vi "EZ430-Chronos - Read Accelerometer.vi"() -> ()   [LabVIEW 2011, in "LVH-EZ430.lvlib"]
doc: "This example demonstrates how to read the accelerometer data from the EZ430-Chronos watch in ACC mode."
uses:
  vi.lib/LabVIEW Hacker/LabVIEW Interface for EZ430-Chronos/LVH-EZ430.lvlib
  vi.lib/LabVIEW Hacker/LabVIEW Interface for EZ430-Chronos/Private/Type Defs/EZ430-Chronos Config.ctl
panel:
  in  "Stop Button":bool
  in  "EZ430-Chronos Config":T1
  out "Accelerations":T2(graph)
  # "EZ430-Chronos Read Accelerometer (ACC) Example\n\nThis example demonstrates how to read the accelerometer data from the EZ430-Chronos watch in ACC mode.\n\nInstructions:\n1. Configure the EZ430-Chronos watch to ACC mode.\n2. Start wireless transmition on the watch.\n3. Select the COM port associated with the EZ430-Chronos USB dongle.\n4. Click the Run Arrow."
  # "EZ430-Chronos Settings"
  # "Acceleration Data"
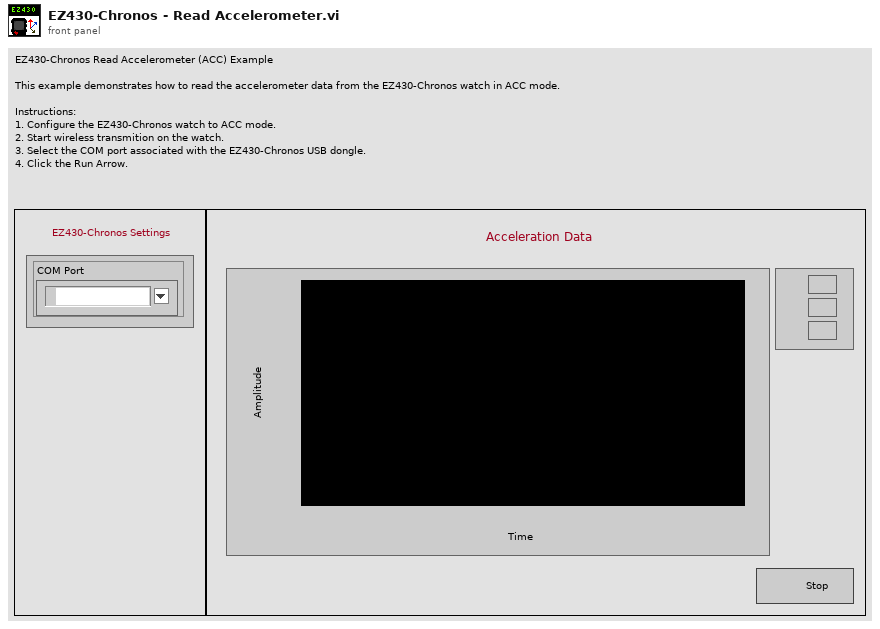
[diagram p1: front panel]
types:
  T1 = typedef "LVH-EZ430.lvlib/EZ430-Chronos Config.ctl" = cluster{"COM Port":refnum<visa-resource-name>}
  T2 = typedef "LVH-EZ430.lvlib/Accelerations.ctl" = cluster{"X Axis":i8, "Y Axis":i8, "Z Axis":i8}
  T3 = typedef "LVH-EZ430.lvlib/EZ430-Chronos Ref.ctl" = cluster{"COM Port":refnum<visa-resource-name>}
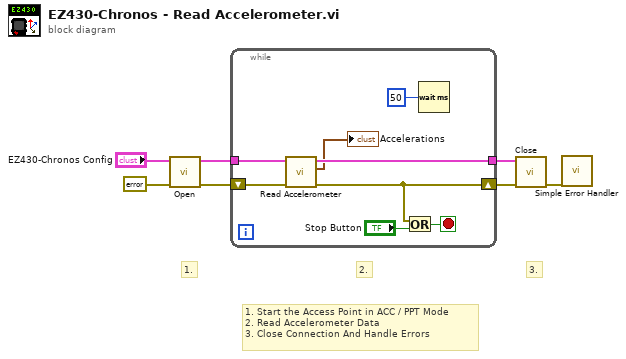
[diagram p0: block diagram]
diagram:
  # "1. Start the Access Point in ACC / PPT Mode\n2. Read Accelerometer Data\n3. Close Connection And Handle Errors"
  # "3."
  # "2."
  # "1."
  n1 = call "Open.vi"("Error In"=errorcluster {"status"=FALSE, "code"=0, "source"=""}, "EZ430-Chronos Config"="EZ430-Chronos Config") -> ("Error Out"=w2:errorcluster, "EZ430-Chronos Ref"=w3:T3)  [unwired: 8 in]
  n2 = while {
    tunnel: w3 -> [w15]
    tunnel: [w13] -> w7
    shift-right: [w10] -> w4
    shift-left: w2 -> [w14]
    stop <- w12 stop-if-true
    n3 = call "Read Accelerometer.vi"("Error In"=w14, "EZ430-Chronos Ref"=w15) -> ("Error Out"=w10:errorcluster, "Accelerations"=→"Accelerations":T2, "EZ430-Chronos Config"=w13:T3)  [unwired: 7 in]
    n4 = Or(x=w10, y="Stop Button") -> (x .or. y?=w12:bool)
    n5 = Wait (ms)(milliseconds to wait=u32 50) -> ()  [unwired: 1 out]
  }
  n6 = call "Close.vi"("Error In"=w4, "EZ430-Chronos Config"=w7) -> ("Error Out"=w1:errorcluster)  [unwired: 9 in]
  n7 = call <vilib>:"Simple Error Handler.vi"("error in (no error)"=w1) -> ()  [unwired: 4 in, 5 out]
